vi "SetPoint.vi"(8 "error in (no error)":errorcluster, 10 "Point":refnum<class "Point.lvclass">, 11 "Square in":refnum<class "Square.lvclass">) -> (0 "error out":errorcluster, 3 "Square out":refnum<class "Square.lvclass">)   [LabVIEW 2021, in "Picture2D.lvlib" / "Square.lvclass"]
uses:
  Square.lvclass
  Rectangle/Rectangle.lvclass
  Point/Point.lvclass
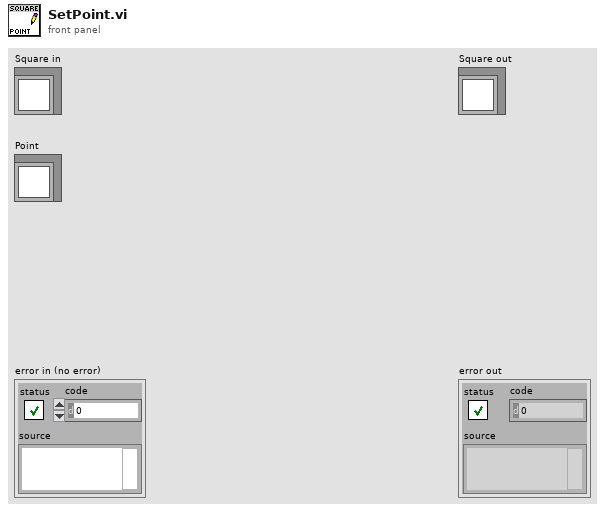
[diagram p1: front panel]
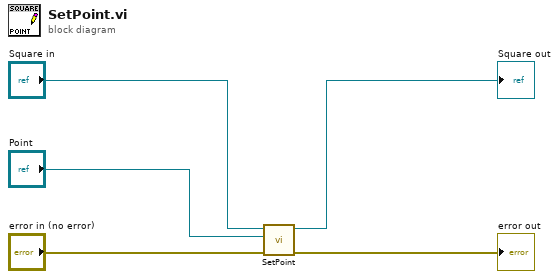
[diagram p0: block diagram]
diagram:
  n1 = call-parent "SetPoint.vi"("error in (no error)"="error in (no error)", "Point"="Point", "Rectangle in"="Square in") -> ("error out"=→"error out":errorcluster, "Rectangle out"=→"Square out":refnum<class "Square.lvclass">)  [unwired: 7 in]
